vi "sub_main_sound.vi"(8 "error in":errorcluster) -> (0 "error out":errorcluster)   [LabVIEW 2019]
uses:
  Ctrl/cmd_common.ctl
  Ctrl/sound-data.ctl
  <vilib>/numeric/Random Number (Range) U64.vi
  <vilib>/numeric/Random Number (Range) I64.vi
  <vilib>/numeric/sub_Random U32.vi
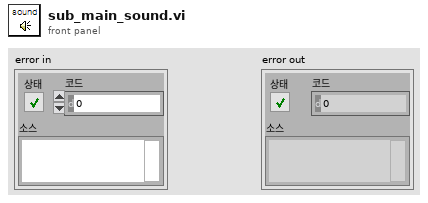
[diagram p1: front panel]
types:
  T1 = enum16{"check", "unlock", "engine", "warning", "msg", "music"}
  T2 = typedef "sound-data.ctl" = cluster{"FN":enum16{"check", "unlock", "engine", "warning", "msg", "music"}, "Data":variant}
  T3 = typedef "cmd_common.ctl" = enum16{"read", "write"}
  T4 = typedef "Sound Output Task ID.ctl" = u32
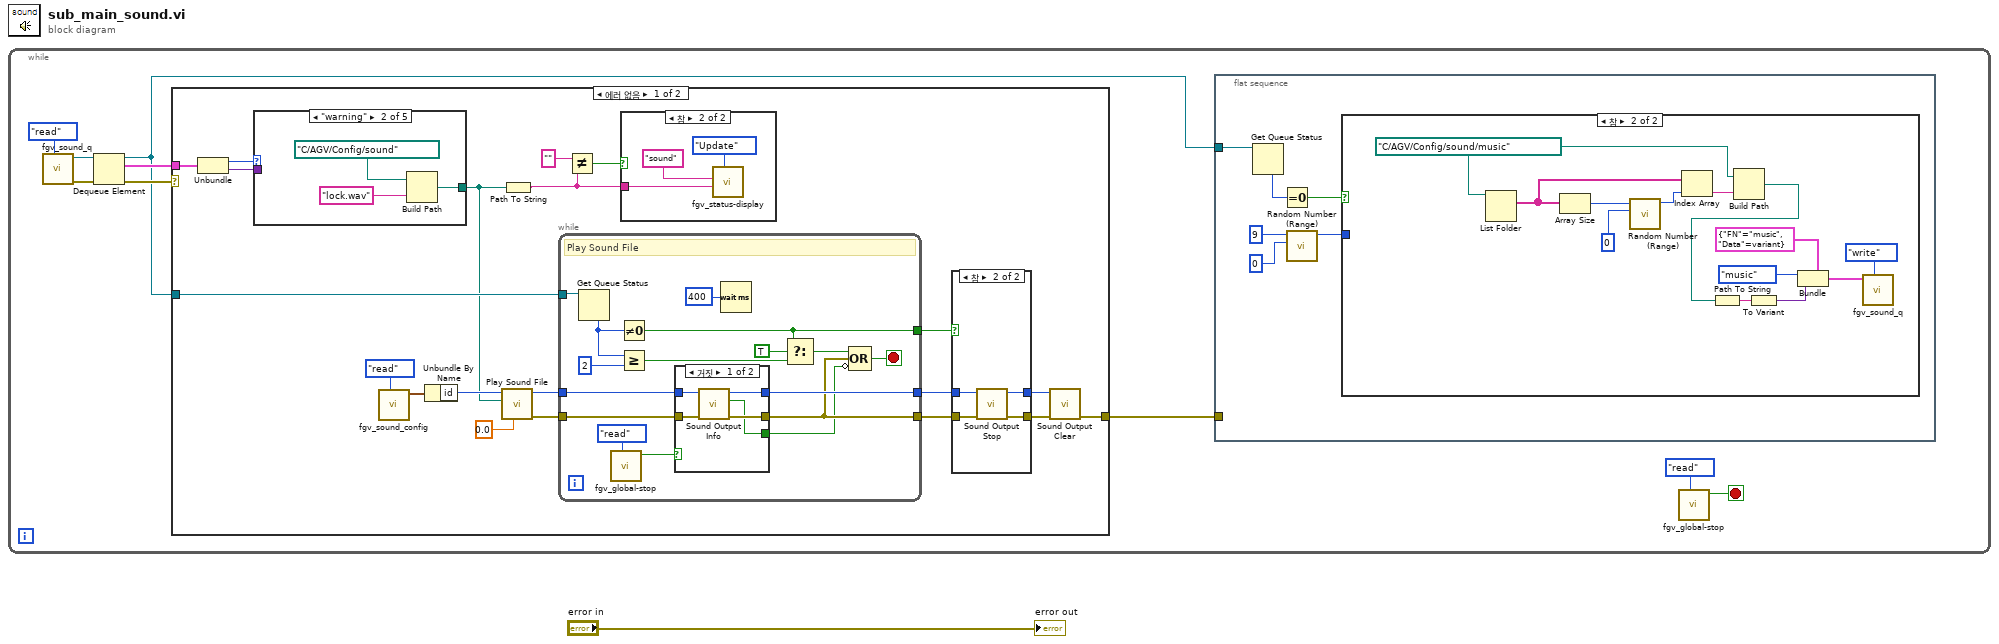
[diagram p0: block diagram]
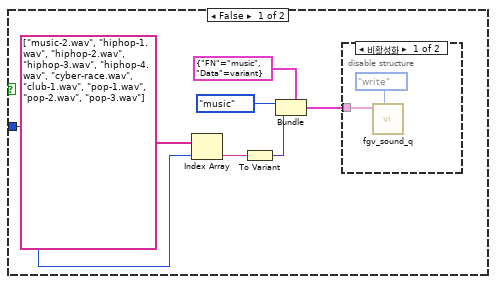
[diagram p2: hidden frame]
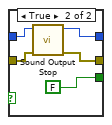
[diagram p6: hidden frame]
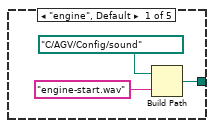
[diagram p7: hidden frame]
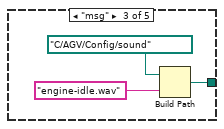
[diagram p8: hidden frame]
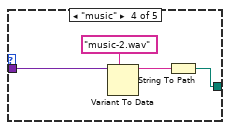
[diagram p9: hidden frame]
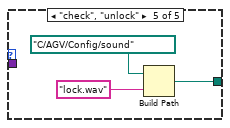
[diagram p10: hidden frame]
diagram:
  n1 = while {
    stop <- w6 stop-if-true
    n2 = call "fgv_sound_q.vi"("cmd"=enum16{"create", "write", "read", "close"}."read") -> ("error out"=w8:errorcluster, "queue out"=w7:refnum<queue>)  [unwired: 9 in]
    n3 = Dequeue Element(queue=w7, error in (no error)=w8) -> (queue out=w2:refnum<queue>, element=w4:T2, error out=w5:errorcluster)  [unwired: 1 in, 1 out]
    n4 = case shown="에러 없음" w5 {
      tunnel: w4 -> [w58 _]
      tunnel: [w51 _] -> w3
      tunnel: w2 -> [w50 _]
      frame No Error {
        n5 = Unbundle(w58) -> ("FN"=w57:T1, "Data"=w42:variant)
        n6 = case shown="\"warning\"" w57 {
          tunnel: w42 -> [_ _ _ w106 _]
          tunnel: [w94 w97 w100 w103 w107] -> w41
          frame "engine", Default {
            n7 = Build Path(base path=path "C:/AGV/Config/sound" ("베이스 경로"), name or relative path="engine-start.wav") -> (appended path=w94:path)
          }
          frame "warning" {
            n8 = Build Path(base path=path "C:/AGV/Config/sound" ("베이스 경로"), name or relative path="lock.wav") -> (appended path=w97:path)
          }
          frame "msg" {
            n9 = Build Path(base path=path "C:/AGV/Config/sound" ("베이스 경로"), name or relative path="engine-idle.wav") -> (appended path=w100:path)
          }
          frame "music" {
            n10 = Variant To Data(type="music-2.wav", Variant=w106) -> (data=w104:string)  [unwired: 1 in, 1 out]
            n11 = String To Path(string=w104) -> (path=w103:path)
          }
          frame "check", "unlock" {
            n12 = Build Path(base path=path "C:/AGV/Config/sound" ("베이스 경로"), name or relative path="lock.wav") -> (appended path=w107:path)
          }
        }
        n13 = call "fgv_sound_config.vi"("cmd"=cmd_common."read") -> ("data out"=w53:cluster{"id":u32})  [unwired: 10 in]
        n14 = Unbundle By Name(w53) -> ("id"=w52:u32)
        n15 = call <vilib>:"Play Sound File.vi"("timeout (sec)"=0.0, "path"=w41, "device ID"=w52) -> ("error out"=w55:errorcluster, "task ID"=w56:T4)  [unwired: 7 in]
        n16 = Path To String(path=w41) -> (string=w40:string)
        n17 = while {
          tunnel: w56 -> [w78]
          tunnel: [w82] -> w47
          tunnel: w55 -> [w79]
          tunnel: [w81] -> w46
          tunnel: w50 -> [w74]
          tunnel: [w71] -> w49
          stop <- w83 stop-if-true
          # "Play Sound File"
          n18 = Get Queue Status(queue=w74) -> (# elements in queue=w73:i32)  [unwired: 2 in, 7 out]
          n19 = call "fgv_global-stop.vi"("cmd"=enum16{"init", "stop", "read"}."read") -> ("val_out"=w75:bool)  [unwired: 10 in]
          n20 = Not Equal To 0?(x=w73) -> (x != 0?=w71:bool)
          n21 = Greater Or Equal?(x=w73, y=2) -> (x >= y?=w70:bool)
          n22 = case shown="거짓" w75 {
            tunnel: w79 -> [w88 w92]
            tunnel: [w87 w90] -> w82
            tunnel: w78 -> [w86 w93]
            tunnel: [w85 w91] -> w81
            tunnel: [w84 FALSE] -> w80
            frame False {
              n23 = call <vilib>:"Sound Output Info.vi"("error in (no error)"=w88, "task ID"=w86) -> ("error out"=w85:errorcluster, "is playing?"=w84:bool, "task ID out"=w87:T4)  [unwired: 6 in, 1 out]
            }
            frame True {
              n24 = call <vilib>:"Sound Output Stop.vi"("error in (no error)"=w92, "task ID"=w93) -> ("error out"=w91:errorcluster, "task ID out"=w90:T4)  [unwired: 8 in]
            }
          }
          n25 = Wait (ms)(milliseconds to wait=u32 400) -> ()  [unwired: 1 out]
          n26 = Select(t=w71, s=TRUE, f=w70) -> (s? t:f=w69:bool)
          n27 = Compound Arithmetic op=OR(w69, w81, invert w80) -> (w83:bool)
        }
        n28 = Not Equal?(x="", y=w40) -> (x != y?=w43:bool)
        n29 = case shown="참" w43 {
          tunnel: w40 -> [_ w59]
          frame False {
          }
          frame True {
            n30 = call "fgv_status-display.vi"("Mode"=enum16{"Initial", "Update", "Clear"}."Update", "detail"=w59, "title"="sound") -> ()  [unwired: 8 in, 1 out]
          }
        }
        n31 = case shown="참" w49 {
          tunnel: [w63 w67] -> w48
          tunnel: w47 -> [w63 w64]
          tunnel: w46 -> [w62 w66]
          tunnel: [w62 w65] -> w45
          frame False {
          }
          frame True {
            n32 = call <vilib>:"Sound Output Stop.vi"("error in (no error)"=w66, "task ID"=w64) -> ("error out"=w65:errorcluster, "task ID out"=w67:T4)  [unwired: 8 in]
          }
        }
        n33 = call <vilib>:"Sound Output Clear.vi"("error in (no error)"=w45, "task ID"=w48) -> ("error out"=w51:errorcluster)  [unwired: 9 in]
      }
      frame Error {
      }
    }
    n34 = flat-sequence {
      tunnel: w2 -> [w16]
      tunnel: w3 -> [_]
      frame #0 {
        n35 = Get Queue Status(queue=w16) -> (# elements in queue=w15:i32)  [unwired: 2 in, 7 out]
        n36 = Equal To 0?(x=w15) -> (x = 0?=w11:bool)
        n37 = call-poly <vilib>:"Random Number (Range).vi"("lower bound (0)"=u64 0, "upper bound (100)"=u64 9) -> ("number"=w12:u64)  [unwired: 9 in]
        n38 = case shown="참" w11 {
          tunnel: w12 -> [w17 _]
          frame False {
            n39 = Index Array(array=string[] ["music-2.wav", "hiphop-1.wav", "hiphop-2.wav", "hiphop-3.wav", "hiphop-4.wav", "cyber-race.wav", "club-1.wav", "pop-1.wav", "pop-2.wav", "pop-3.wav"], index=w17) -> (element=w18:string)
            n40 = To Variant(anything=w18) -> (Variant=w20:variant)
            n41 = Bundle(cluster=T2 {"FN"=enum."music", "Data"=variant} ("data"), "FN"=T1."music", "Data"=w20) -> (w21:T2)
            n42 = disable-structure shown="비활성화" {
              disable-tunnel: w21 -> [w24 _]
              frame Disabled {
                n43 = call "fgv_sound_q.vi"("cmd"=enum16{"create", "write", "read", "close"}."write", "data"=w24) -> ()  [unwired: 8 in, 2 out]
              }
              frame Enabled {
              }
            }
          }
          frame True {
            w26 = path "C:/AGV/Config/sound/music" ("베이스 경로")
            n44 = List Folder(path=w26) -> (filenames=w36:string[])  [unwired: 3 in, 3 out]
            n45 = Array Size(array=w36) -> (size(s)=w38:i32)
            n46 = call-poly <vilib>:"Random Number (Range).vi"("lower bound (-100)"=i64 0, "upper bound (100)"=w38) -> ("number"=w35:i64)  [unwired: 9 in]
            n47 = Index Array(array=w36, index=w35) -> (element=w34:string)
            n48 = Build Path(base path=w26, name or relative path=w34) -> (appended path=w28:path)
            n49 = Path To String(path=w28) -> (string=w27:string)
            n50 = To Variant(anything=w27) -> (Variant=w29:variant)
            n51 = Bundle(cluster=T2 {"FN"=enum."music", "Data"=variant} ("data"), "FN"=T1."music", "Data"=w29) -> (w30:T2)
            n52 = call "fgv_sound_q.vi"("cmd"=enum16{"create", "write", "read", "close"}."write", "data"=w30) -> ()  [unwired: 8 in, 2 out]
          }
        }
      }
    }
    n53 = call "fgv_global-stop.vi"("cmd"=enum16{"init", "stop", "read"}."read") -> ("val_out"=w6:bool)  [unwired: 10 in]
  }
  "error out" <- "error in"
